vi "DAQ_Assistant_Ref_Signal.vi"(9 "stop (F)":bool, 10 "rate":dbl=1000.0) -> (2 "data 2":dynamicdata(graph) caption="data")   [LabVIEW 2018]
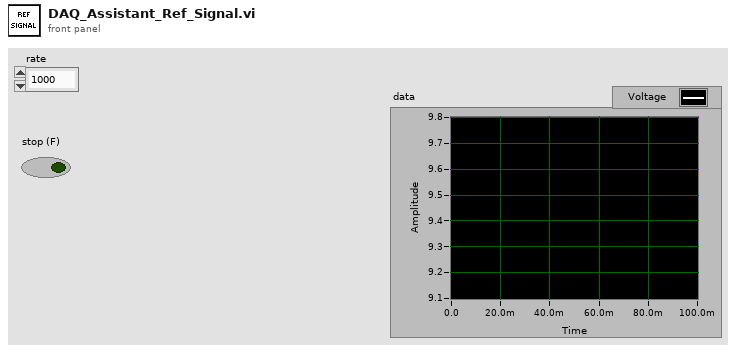
[diagram p1: front panel]
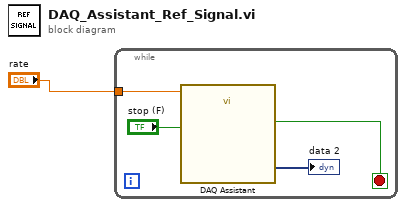
[diagram p0: block diagram]
diagram:
  n1 = while {
    tunnel: "rate" -> [w2]
    stop <- w4 stop-if-true
    n2 = call "DAQ Assistant"("rate"=w2, "stop (F)"="stop (F)") -> ("data"=→"data 2":dynamicdata, "stopped"=w4:bool)  [unwired: 14 in, 2 out]
  }
